vi "ProcessPath.vi"(8 "error in (no error)":errorcluster, 11 "path in":path) -> (0 "error out":errorcluster, 2 "Type":string, 3 "path out":path, 4 "Is Directory?":bool, 5 "File/Folder name":string)   [LabVIEW 2017]
uses:
  <vilib>/Utility/error.llb/Error Cluster From Error Code.vi
  <vilib>/ErrorRing/Error Ring.xnode
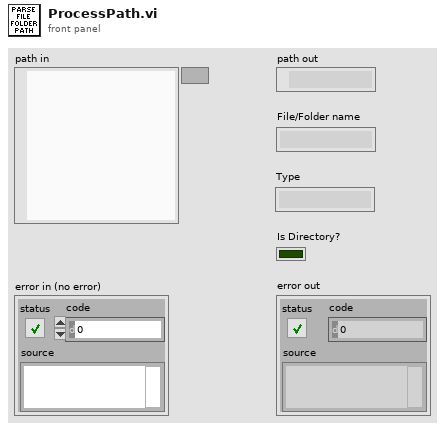
[diagram p1: front panel]
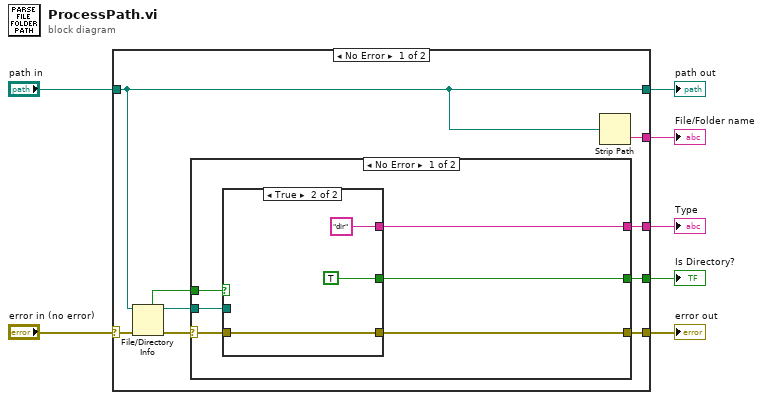
[diagram p0: block diagram]
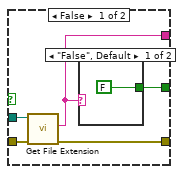
[diagram p2: hidden frame]
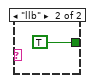
[diagram p3: hidden frame]
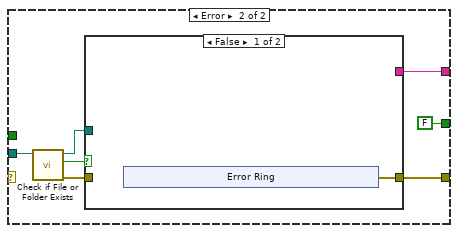
[diagram p4: hidden frame]
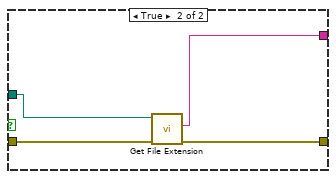
[diagram p5: hidden frame]
diagram:
  n1 = case shown="No Error" "error in (no error)" {
    selector: "error in (no error)" -> [w14 w50]
    tunnel: [w10 w49] -> w6
    tunnel: "path in" -> [w10 w49]
    tunnel: [w16 _] -> w5
    tunnel: [w15 w50] -> w4
    tunnel: [w9 _] -> w3
    tunnel: [w8 _] -> w2
    frame No Error {
      n2 = File/Directory Info(path=w10, error in=w14) -> (path out=w11:path, directory=w12:bool, error out=w13:errorcluster)  [unwired: 4 out]
      n3 = case shown="No Error" w13 {
        selector: w13 -> [w20 _]
        tunnel: [w22 FALSE] -> w16
        tunnel: [w21 w35] -> w15
        tunnel: w12 -> [w19 _]
        tunnel: w11 -> [w18 w39]
        tunnel: [w17 w33] -> w8
        frame No Error {
          n4 = case shown="True" w19 {
            tunnel: w18 -> [w27 _]
            tunnel: [w26 TRUE] -> w22
            tunnel: [w24 w31] -> w21
            tunnel: w20 -> [w25 w31]
            tunnel: [w23 "dir"] -> w17
            frame False {
              n5 = call <vilib>:"Get File Extension.vi"("error in (no error)"=w25, "file"=w27) -> ("error out"=w24:errorcluster, "lowercase file extension"=w23:string)  [unwired: 5 in, 3 out]
              n6 = case shown="\"False\", Default" w23 {
                tunnel: [FALSE TRUE] -> w26
                frame "False", Default {
                }
                frame "llb" {
                }
              }
            }
            frame True {
            }
          }
        }
        frame Error {
          n7 = call <vilib>:"Check if File or Folder Exists.vi"("path"=w39) -> ("error out"=w36:errorcluster, "file or folder exists?"=w37:bool, "dup path"=w34:path)  [unwired: 8 in]
          n8 = case shown="False" w37 {
            tunnel: w36 -> [_ w48]
            tunnel: [w40 w47] -> w35
            tunnel: w34 -> [_ w46]
            tunnel: [_ w45] -> w33
            frame False {
              n9 = xnode "Error Ring"() -> ("error out"=w40:errorcluster)
            }
            frame True {
              n10 = call <vilib>:"Get File Extension.vi"("error in (no error)"=w48, "file"=w46) -> ("error out"=w47:errorcluster, "lowercase file extension"=w45:string)  [unwired: 5 in, 3 out]
            }
          }
        }
      }
      n11 = Strip Path(path=w10) -> (name=w9:string)  [unwired: 1 out]
    }
    frame Error {
    }
  }
  "path out" <- w6
  "Is Directory?" <- w5
  "error out" <- w4
  "File/Folder name" <- w3
  "Type" <- w2
